vi "Get Trench Angle.vi"(1 "Distance 2":dbl, 3 "Distance 1":dbl) -> (0 "Current Angle":dbl)   [LabVIEW 2019]
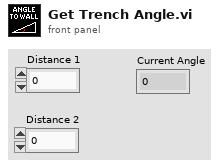
[diagram p1: front panel]
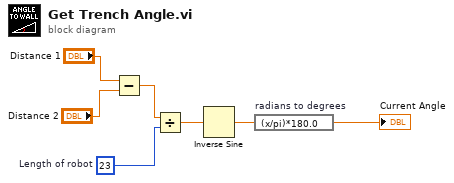
[diagram p0: block diagram]
diagram:
  w4 = 23  # Length of robot
  n1 = Subtract(x="Distance 1", y="Distance 2") -> (x-y=w5:dbl)
  n2 = Divide(x=w5, y=w4) -> (x/y=w3:dbl)
  n3 = Inverse Sine(1:w3) -> (0:w2:dbl)
  n4 = expression code="(x/pi)*180.0" "radians to degrees"(w2) -> (→"Current Angle":dbl)
